vi "Initialize With Dialog.vi"(8 "error in (no error)":errorcluster, 11 "Sound Player in":refnum<class "Sound Card.lvclass">) -> (0 "error out":errorcluster, 2 "Cancelled?":bool, 3 "Sound Player out":refnum<class "Sound Card.lvclass">)   [LabVIEW 2016, in "Sound Card.lvclass"]
doc: "Show configuration dialog for the Sound Card."
uses:
  Sound Card.lvclass
  <vilib>/sound2/lvsound2.llb/Sound Data Format.ctl
  <vilib>/sound2/lvsound2.llb/Sampling Mode.ctl
  Sound Card.lvclass/Sound Card.ctl
  <vilib>/sound2/lvsound2.llb/Sound Output Set Volume (Single).vi
panel:
  in  "Sound Format":T1={"sample rate (S/s)"=44100.0, "number of channels"=2, "bits per sample"=16}
  in  "Volume":dbl(slide)=70.40816326530613 scale=0.0..100.0
  in  "Number of Samples/ch":i32=5000
  in  "Device ID":u32
  in  "Cancel":bool
  in  "OK":bool
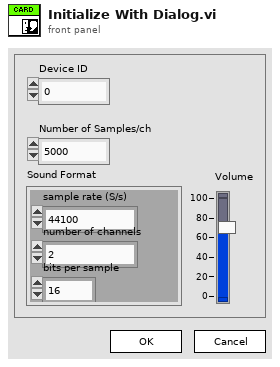
[diagram p1: front panel]
types:
  T1 = typedef "Sound Data Format.ctl" = cluster{"sample rate (S/s)":dbl, "number of channels":i32, "bits per sample":i32}
  T2 = typedef "Sampling Mode.ctl" = i32
  T3 = typedef "Sound Output Task ID.ctl" = u32
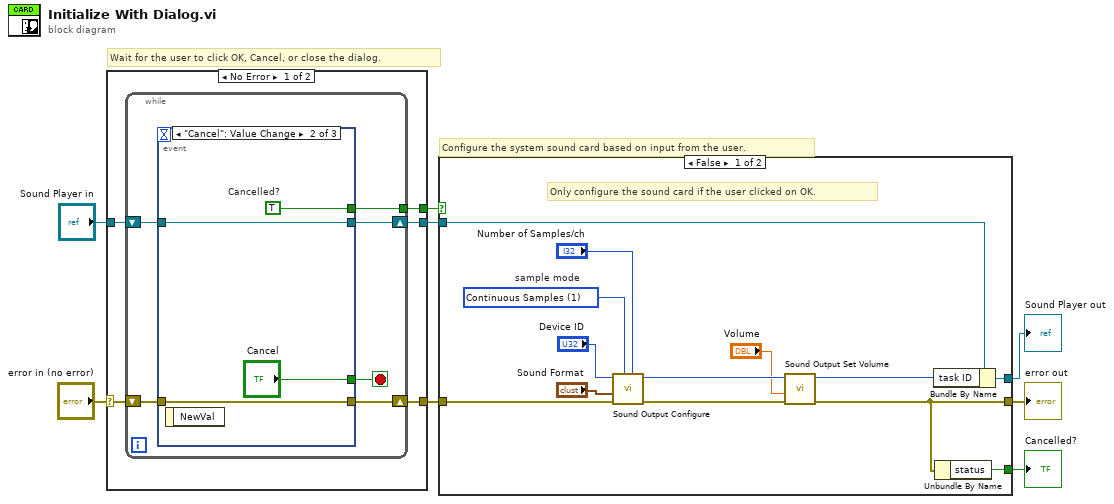
[diagram p0: block diagram]
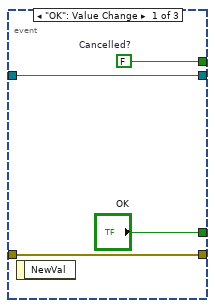
[diagram p3: hidden frame]
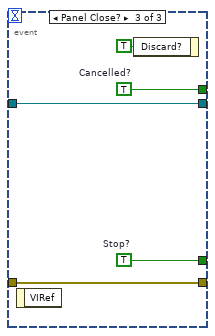
[diagram p4: hidden frame]
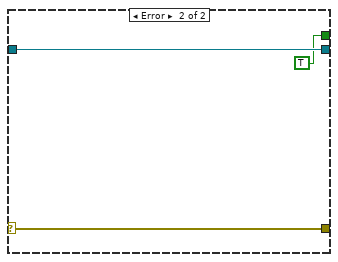
[diagram p5: hidden frame]
diagram:
  # "Configure the system sound card based on input from the user."
  # "Wait for the user to click OK, Cancel, or close the dialog."
  n1 = case shown="No Error" "error in (no error)" {
    selector: "error in (no error)" -> [w11 w35]
    tunnel: [w13 TRUE ("Cancelled?")] -> w6
    tunnel: [w10 w35] -> w5
    tunnel: [w12 w34] -> w3
    tunnel: "Sound Player in" -> [w9 w34]
    frame No Error {
      n2 = while {
        tunnel: [w18] -> w13
        shift-right: [w17] -> w12
        shift-left: w9 -> [w16]
        shift-right: [w14] -> w10
        shift-left: w11 -> [w15]
        stop <- w19 stop-if-true
        n3 = event shown="[1] \"Cancel\": Value Change" {
          selector: _ -> [_ _ _]
          dyn-events: _ -> [_ _ _]
          timeout: _ -> [_ _ _]
          tunnel: ["OK" "Cancel" w31] -> w19
          tunnel: [w23 w27 w30] -> w18
          tunnel: [w21 w25 w29] -> w17
          tunnel: w16 -> [w21 w25 w29]
          tunnel: w15 -> [w20 w24 w28]
          tunnel: [w20 w24 w28] -> w14
          event "OK": Value Change {
            w23 = FALSE  # Cancelled?
            n4 = event-data() -> ()  [unwired: 1 in, 1 out]
          }
          event "Cancel": Value Change {
            w27 = TRUE  # Cancelled?
            n5 = event-data() -> ()  [unwired: 1 in, 1 out]
          }
          event Panel Close? {
            w30 = TRUE  # Cancelled?
            w31 = TRUE  # Stop?
            n6 = event-data() -> ()  [unwired: 1 in, 1 out]
            n7 = event-data("Discard?"=TRUE) -> ()  [unwired: 1 in, 1 out]
          }
        }
      }
    }
    frame Error {
    }
  }
  n8 = case shown="False" w6 {
    selector: w6 -> [_ w49]
    tunnel: w5 -> [w48 w50]
    tunnel: [w37 w50] -> w4
    tunnel: w3 -> [w40 w51]
    tunnel: [w38 w51] -> w2
    tunnel: [w36 w49] -> w1
    frame False {
      w45 = T2 1 items=["Finite Samples", "Continuous Samples"]  # sample mode
      # "Only configure the sound card if the user clicked on OK."
      n9 = call <vilib>:"Sound Output Configure.vi"("number of samples/ch"="Number of Samples/ch", "sample mode"=w45, "error in (no error)"=w48, "sound format"="Sound Format", "device ID"="Device ID") -> ("error out"=w43:errorcluster, "task ID"=w42:T3)  [unwired: 5 in]
      n10 = call-poly <vilib>:"Sound Output Set Volume.vi"("error in (no error)"=w43, "volume"="Volume", "task ID"=w42) -> ("error out"=w37:errorcluster, "task ID out"=w39:T3)  [unwired: 7 in]
      n11 = Bundle By Name(cluster=w40, "task ID"=w39) -> (w38:refnum<class "Sound Card.lvclass">)
      n12 = Unbundle By Name(w37) -> ("status"=w36:bool)
    }
    frame True {
      # "The user clicked on Cancel or closed the dialog."
    }
  }
  "Cancelled?" <- w1
  "Sound Player out" <- w2
  "error out" <- w4
